vi "Memory.Pointer.Read.All.In Place.vi"   [LabVIEW 2016, in "LabVIEW Memory Manager.lvlib" / "Memory.Pointer.lvclass"]
uses:
  Memory.Pointer.lvclass
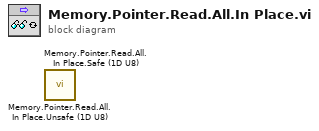
[diagram p0: block diagram]
diagram:
  n1 = call "Memory.Pointer.Read.All.In Place.Unsafe (1D U8).vi"() -> ()  [unwired: 9 in, 3 out]
  n2 = call "Memory.Pointer.Read.All.In Place.Safe (1D U8).vi"() -> ()  [unwired: 9 in, 3 out]
